vi "MCfrontPanel.vi"() -> ()   [LabVIEW 2014]
uses:
  Path.ctl
panel:
  in  "Tab Control":enum32{"Setup", "Debug", "Process", "Review"}(tab)
  in  "Next Button":bool
  in  "Previous Button":bool
  in  "Broken Path":dbl
  in  "Exceed Mirror Velocity":dbl
  in  "Number Errors":dbl
  in  "Machine":T1(tab)
  in  "Piston Controller":u16(ring) items=["Newport", "National Instruments"]
  in  "Mirrors And Laser":u16(ring) items=["Choose...", "MachineLogger", "MachineSimulator"]
  out "Bed Size":cluster{"X":dbl, "Y":dbl}
  out "MaxPower":dbl
  out "MaxSpeed":dbl
  in  "Overhand Speed (mm/s)":dbl
  in  "Mirror Speed (mm/s)":dbl
  in  "Record Images?":bool
  out "DLL_Location":path=path "C:/Users/guss2/Desktop/GVI/Git/LVslicer/MachineController/DLL"
  in  "Machine Preset":u16(ring) items=["Fraunhofer", "EOS", "Custom 1", "My Special Settings"]
  out "File":path
  out "File Stats":T2
  in  "Layer Display":dbl
  out "Yplot":dbl[](graph)
  out "Xplot":dbl[](graph)
  out "Layer":cluster{dbl[], dbl[]}(graph)
  in  "Load SCAN":bool
  in  "Beam Location":cluster{"X":dbl, "Y":dbl}
  in  "Power (W)":dbl
  in  "Laser":bool
  out "Remaining Time":string
  out "Laser Power":dbl
  out "Mirror Y":dbl
  out "Mirror X":dbl
  out "Number Errors":dbl
  out "Layer":dbl(slide) scale=0.0..1036.0
  out "3D Picture":refnum<vi>(3d-picture)
  out "ETA":timestamp
  out "Log":string
  in  "Stop Button":bool
  in  "Pause Button":bool
  in  "Play Button":bool
  out "Elapsed Time":string
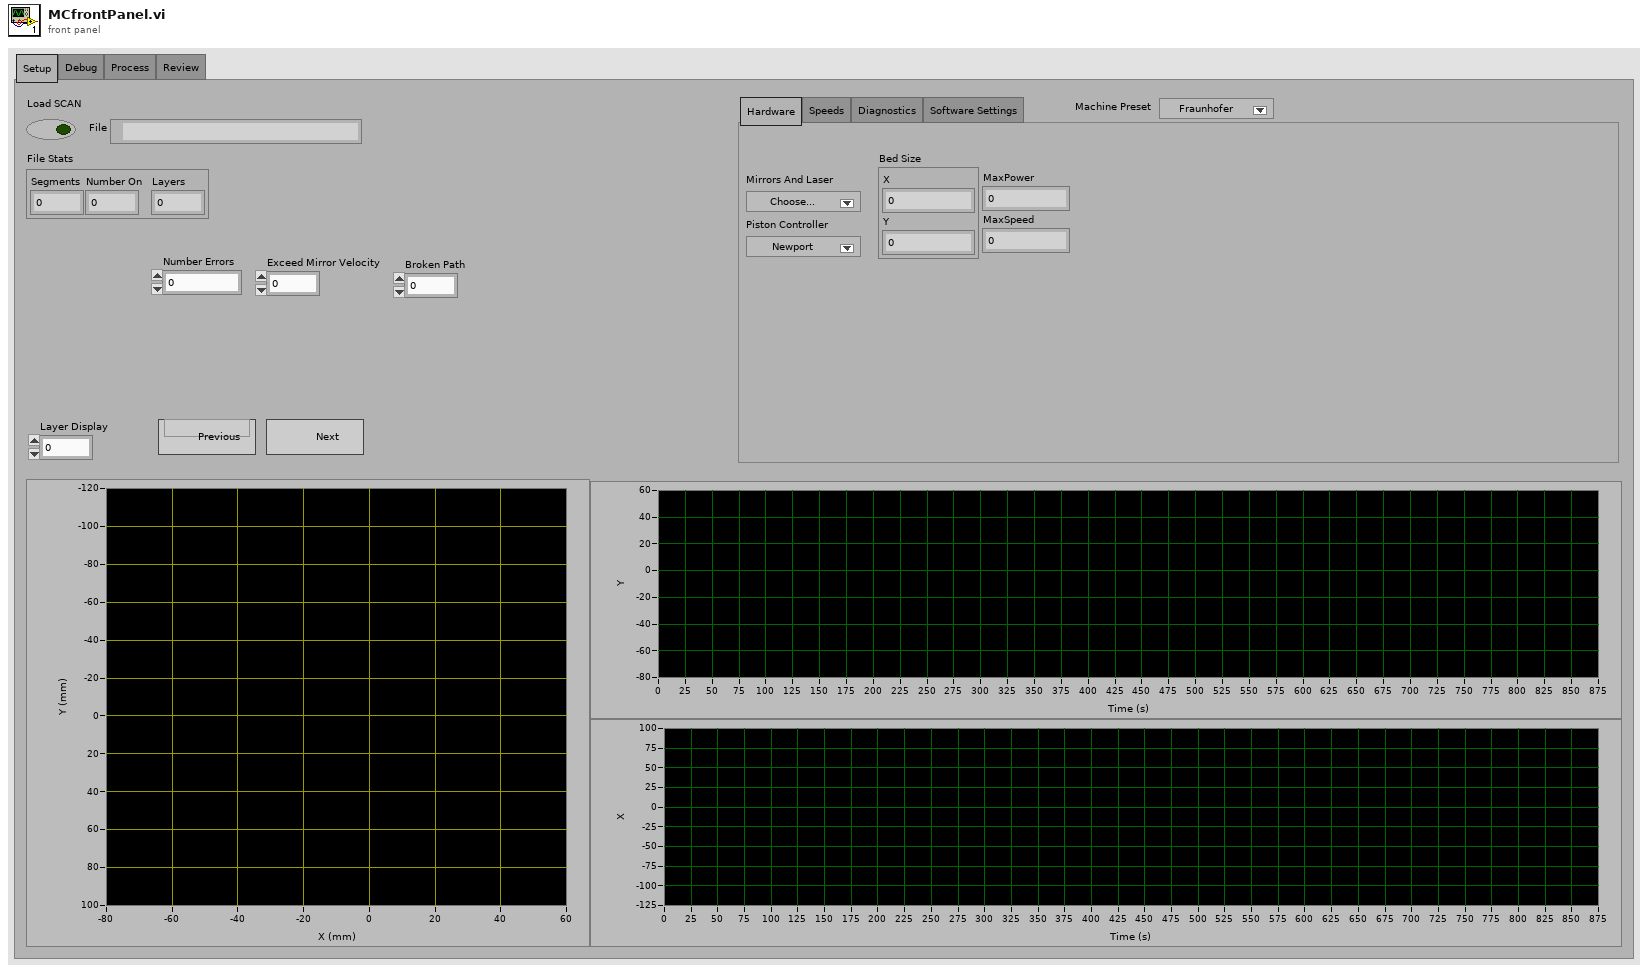
[diagram p1: front panel]
types:
  T1 = enum32{"Hardware", "Speeds", "Diagnostics", "Software Settings"}
  T2 = cluster{"Segments":dbl, "Number On":dbl, "Layers":dbl}
  T3 = typedef "Path.ctl" = cluster{"X":dbl, "Y":dbl, "OnOff":bool}[]
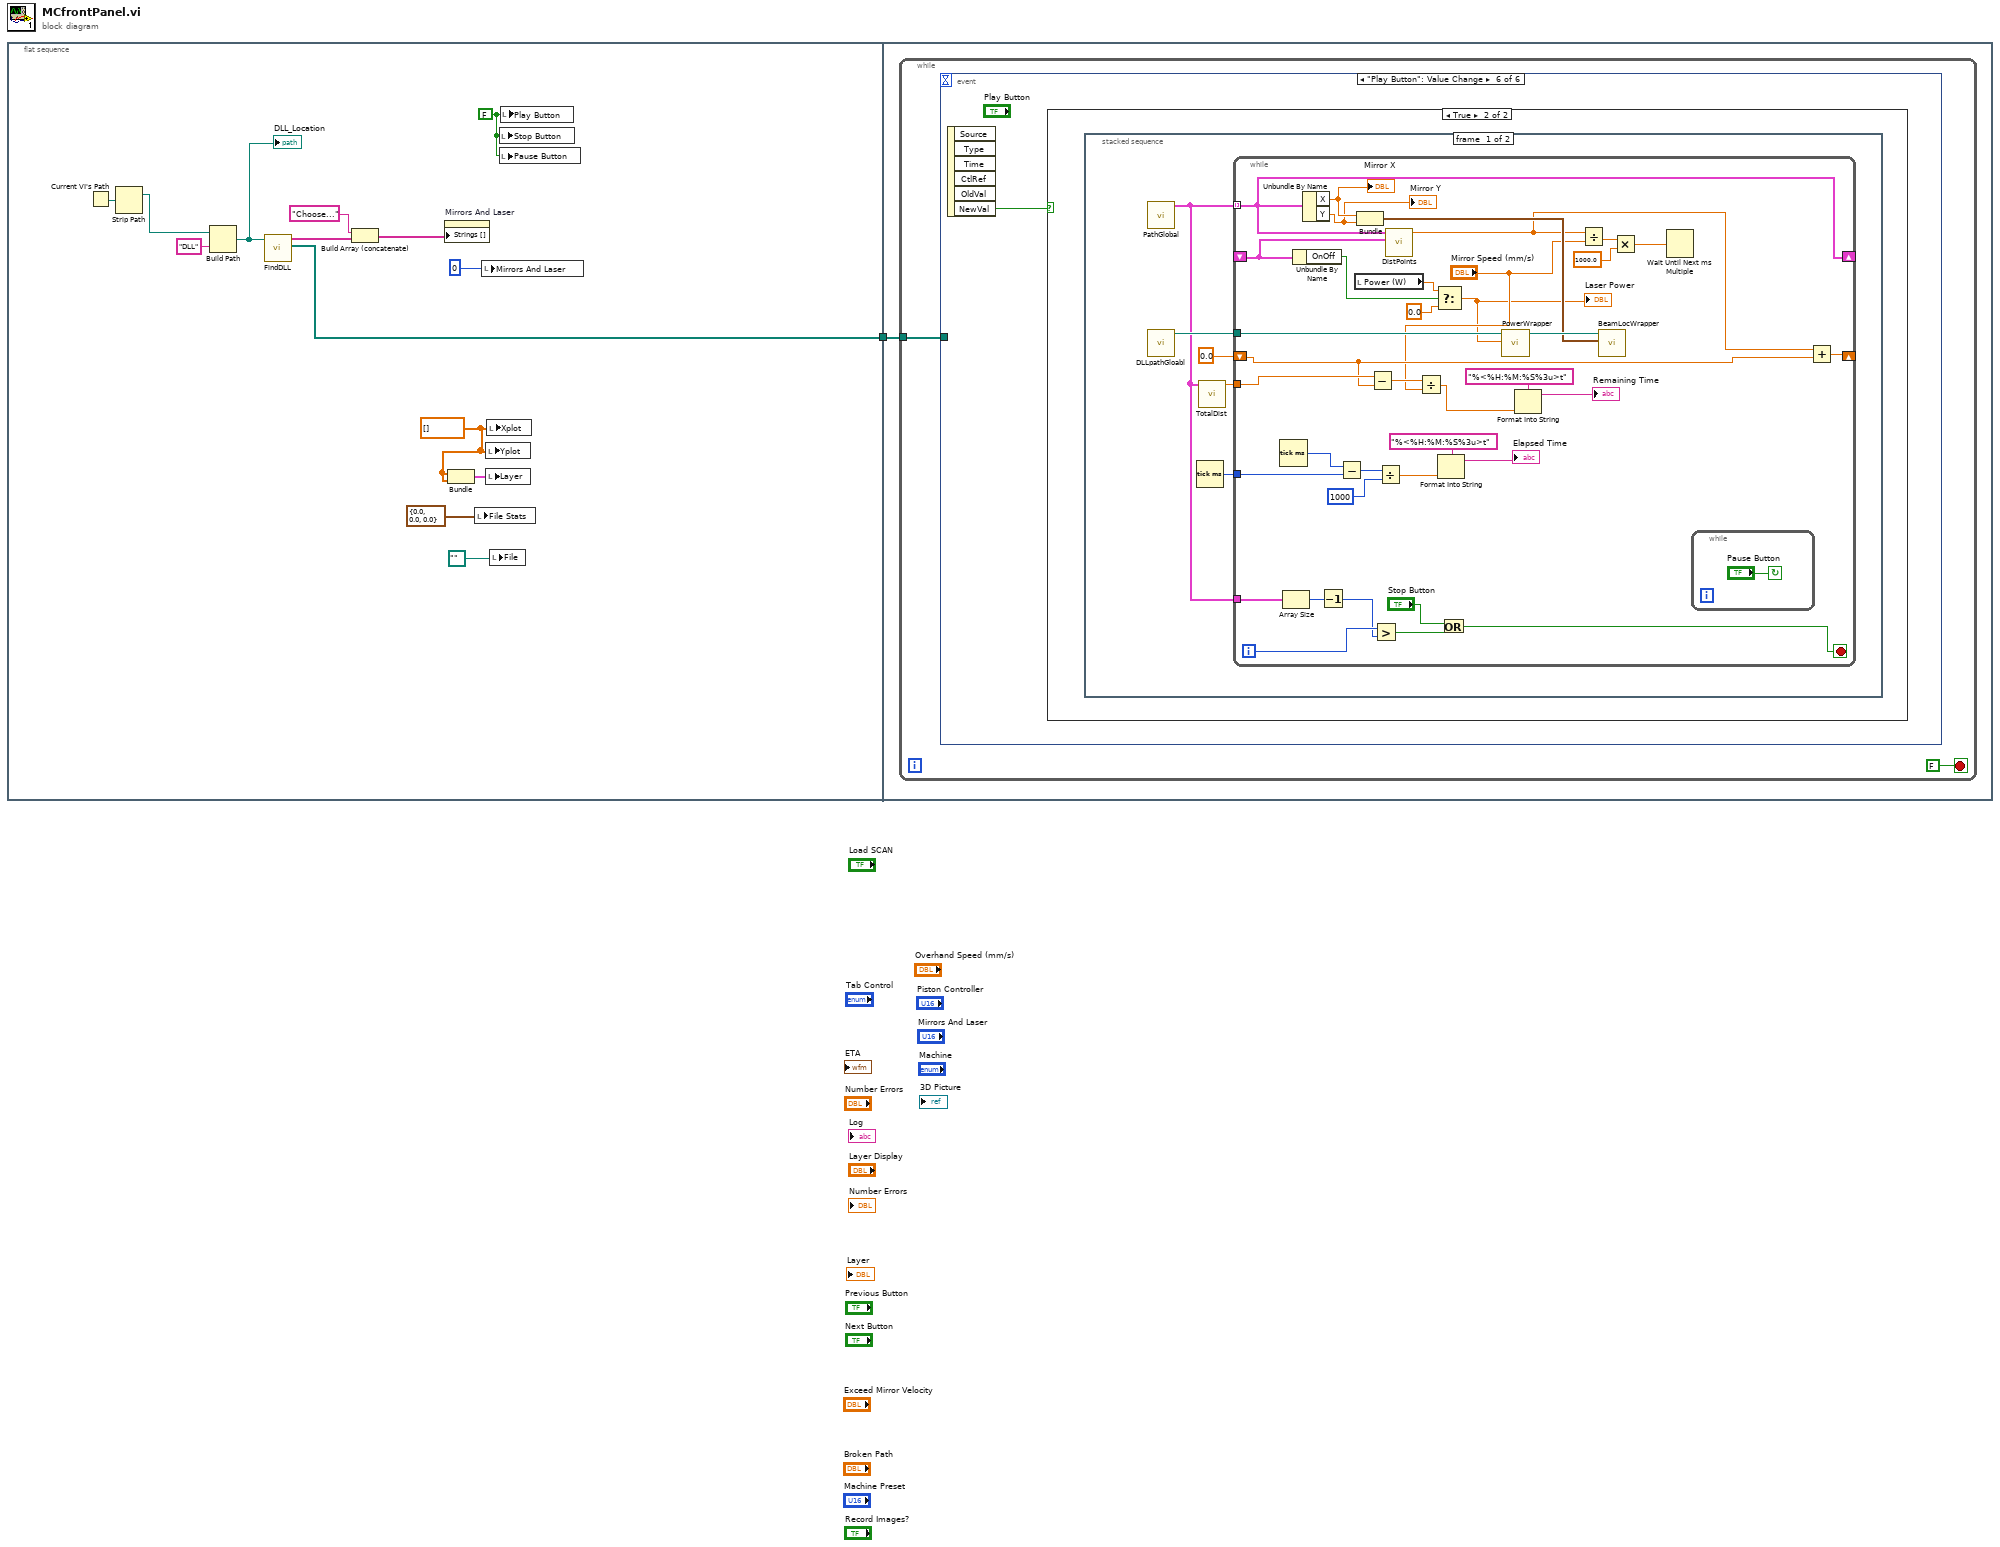
[diagram p0: block diagram]
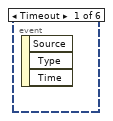
[diagram p2: hidden frame]
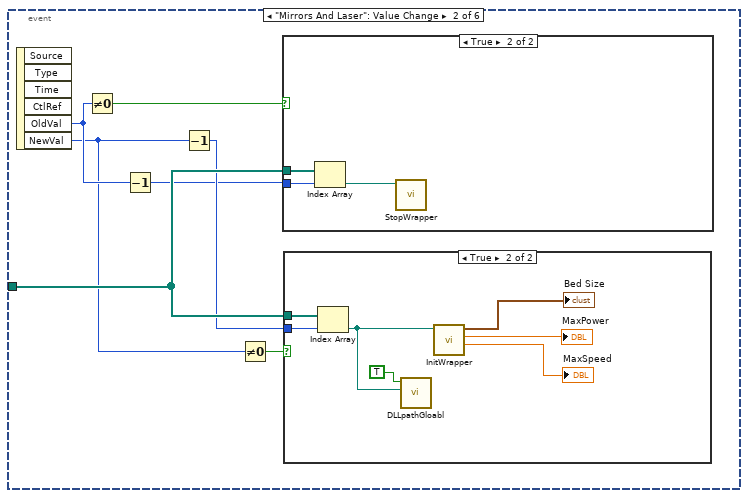
[diagram p3: hidden frame]
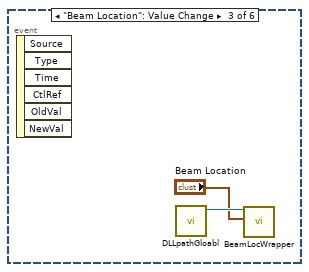
[diagram p6: hidden frame]
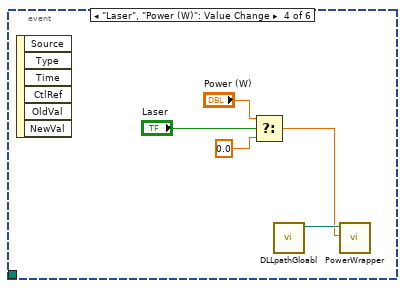
[diagram p7: hidden frame]
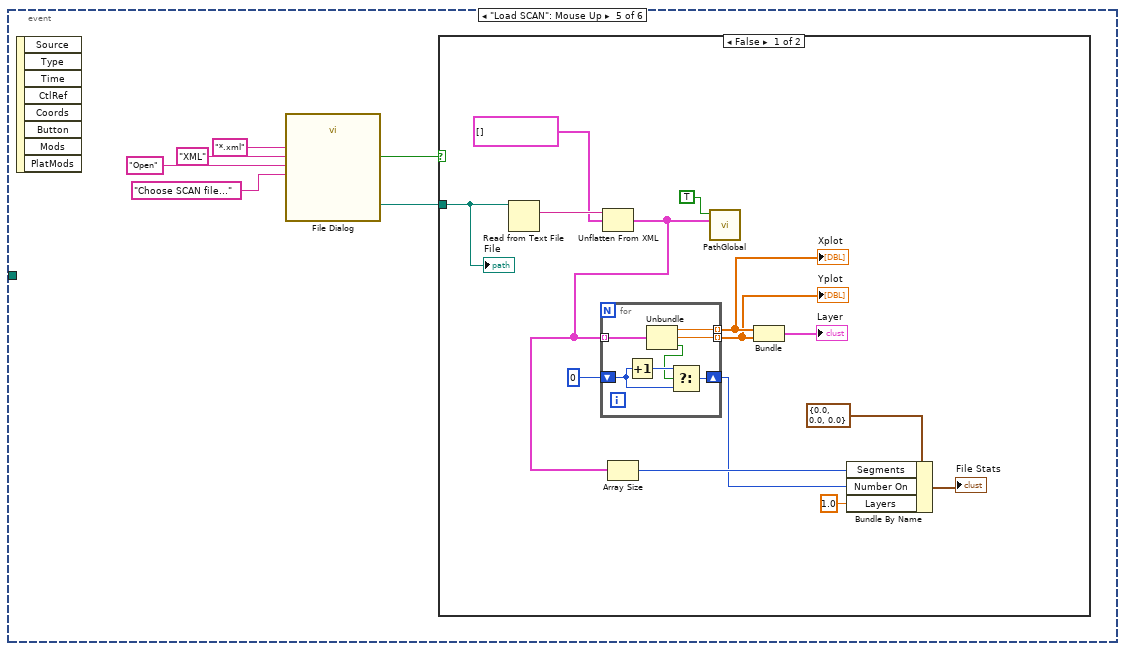
[diagram p8: hidden frame]
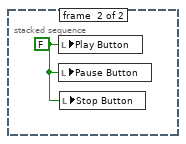
[diagram p11: hidden frame]
diagram:
  n1 = flat-sequence {
    tunnel: [w11] -> w1
    tunnel: w1 -> [w16]
    frame #0 {
      w9 = dbl[] [] ("Xplot")
      w10 = FALSE ("Play Button")
      n2 = Current VI's Path() -> (path=w3:path)
      n3 = Strip Path(path=w3) -> (stripped path=w2:path)  [unwired: 1 out]
      n4 = Build Path(base path=w2, name or relative path="DLL") -> (appended path=w4:path)
      "DLL_Location" <- w4
      n5 = call "FindDLL.vi"("DLL_Location"=w4) -> ("DLLfilepaths"=w11:path[], "DLLnames"=w14:string[])  [unwired: 9 in]
      n6 = Build Array (concatenate)("Choose..." ("filename without extension"), w14) -> (w13:string[])
      n7 = property on="Mirrors And Laser" class="Ring (strict)"("Strings []"=w13) -> ()  [unwired: 2 in, 2 out]
      n8 = Bundle("Xplot"=w9, "Xplot"=w9) -> (w8:cluster{"Xplot":dbl[], "Xplot":dbl[]})  [unwired: 1 in]
      n9 = local write "File Stats"(T2 {"Segments"=0.0, "Number On"=0.0, "Layers"=0.0} ("File Stats")) -> ()
      n10 = local write "Mirrors And Laser"(0) -> ()
      n11 = local write "Yplot"(w9) -> ()
      n12 = local write "Layer"(w8) -> ()
      n13 = local write "Xplot"(w9) -> ()
      n14 = local write "File"(path "" ("File")) -> ()
      n15 = local write "Stop Button"(w10) -> ()
      n16 = local write "Pause Button"(w10) -> ()
      n17 = local write "Play Button"(w10) -> ()
    }
    frame #1 {
      n18 = while {
        tunnel: w16 -> [w17]
        stop <- FALSE stop-if-true
        n19 = event shown="[5] \"Play Button\": Value Change" {
          selector: _ -> [_ _ _ _ _ _]
          dyn-events: _ -> [_ _ _ _ _ _]
          timeout: _ -> [_ _ _ _ _ _]
          tunnel: w17 -> [_ w24 _ _ _ _]
          event Timeout {
            n20 = event-data() -> ()  [unwired: 1 in, 3 out]
          }
          event "Mirrors And Laser": Value Change {
            n21 = event-data() -> ("OldVal"=w21:u16, "NewVal"=w19:u16)  [unwired: 1 in, 4 out]
            n22 = Not Equal To 0?(x=w21) -> (x != 0?=w25:bool)
            n23 = Decrement(x=w21) -> (x-1=w20:u16)
            n24 = Decrement(x=w19) -> (x-1=w22:u16)
            n25 = Not Equal To 0?(x=w19) -> (x != 0?=w23:bool)
            n26 = case shown="True" w25 {
              tunnel: w24 -> [_ w35]
              tunnel: w20 -> [_ w34]
              frame False {
              }
              frame True {
                n27 = Index Array(array=w35, index=w34) -> (element=w33:path)
                n28 = call "StopWrapper.vi"("DLLpath"=w33) -> ()  [unwired: 11 in]
              }
            }
            n29 = case shown="True" w23 {
              tunnel: w22 -> [_ w32]
              tunnel: w24 -> [_ w28]
              frame False {
              }
              frame True {
                n30 = Index Array(array=w28, index=w32) -> (element=w26:path)
                n31 = call "DLLpathGloabl.vi"("DLLpath"=w26, "Set/Get"=TRUE) -> ()  [unwired: 9 in, 1 out]
                n32 = call "InitWrapper.vi"("DLLpath"=w26) -> ("MaxSpeed"=→"MaxSpeed":dbl, "MaxPower"=→"MaxPower":dbl, "Bed Size"=→"Bed Size":cluster{"X":dbl, "Y":dbl})  [unwired: 8 in]
              }
            }
          }
          event "Beam Location": Value Change {
            n33 = event-data() -> ()  [unwired: 1 in, 6 out]
            n34 = call "DLLpathGloabl.vi"() -> ("PathOut"=w37:path)  [unwired: 11 in]
            n35 = call "BeamLocWrapper.vi"("Beam Location"="Beam Location", "DLLpath"=w37) -> ()  [unwired: 10 in]
          }
          event "Laser", "Power (W)": Value Change {
            n36 = event-data() -> ()  [unwired: 1 in, 6 out]
            n37 = Select(t="Power (W)", s="Laser", f=0.0) -> (s? t:f=w41:dbl)
            n38 = call "DLLpathGloabl.vi"() -> ("PathOut"=w42:path)  [unwired: 11 in]
            n39 = call "PowerWrapper.vi"("Power"=w41, "DLLpath"=w42) -> ()  [unwired: 9 in, 1 out]
          }
          event "Load SCAN": Mouse Up {
            n40 = event-data() -> ()  [unwired: 1 in, 8 out]
            n41 = call "File Dialog"("prompt"="Choose SCAN file...", "button label"="Open", "pattern (all files)"="*.xml", "pattern label"="XML") -> ("selected path"=w43:path, "cancelled"=w44:bool)  [unwired: 8 in, 2 out]
            n42 = case shown="False" w44 {
              tunnel: w43 -> [w58 _]
              frame False {
                n43 = Read from Text File(file (use dialog)=w58) -> (text=w62:string)  [unwired: 3 in, 3 out]
                n44 = Unflatten From XML(xml string=w62, type=T3 [] ("PathOut")) -> (value=w56:T3)  [unwired: 1 in, 1 out]
                n45 = for {
                  tunnel: w56 -> [w69] mode=indexing
                  tunnel: [w68] -> w50 mode=indexing
                  tunnel: [w67] -> w49 mode=indexing
                  shift-right: [w66] -> w52
                  shift-left: 0 -> [w64]
                  n46 = Increment(x=w64) -> (x+1=w65:i32)
                  n47 = Unbundle(w69) -> ("X"=w68:dbl, "Y"=w67:dbl, "OnOff"=w63:bool)
                  n48 = Select(t=w65, s=w63, f=w64) -> (s? t:f=w66:i32)
                }
                "Xplot" <- w50
                "Yplot" <- w49
                n49 = Array Size(array=w56) -> (size(s)=w53:i32)
                n50 = call "PathGlobal.vi"("Path"=w56, "Set/Get"=TRUE) -> ()  [unwired: 9 in, 1 out]
                n51 = Bundle(w50, w49) -> (→"Layer":cluster{dbl[], dbl[]})  [unwired: 1 in]
                n52 = Bundle By Name(cluster=T2 {"Segments"=0.0, "Number On"=0.0, "Layers"=0.0} ("File Stats"), "Segments"=w53, "Number On"=w52, "Layers"=1.0) -> (→"File Stats":T2)
                "File" <- w58
              }
              frame True {
              }
            }
          }
          event "Play Button": Value Change {
            n53 = event-data() -> ("NewVal"=w70:bool)  [unwired: 1 in, 5 out]
            n54 = case shown="True" w70 {
              frame False {
              }
              frame True {
                n55 = stacked-sequence {
                  frame #0 {
                    n56 = call "PathGlobal.vi"() -> ("PathOut"=w74:T3)  [unwired: 11 in]
                    n57 = call "DLLpathGloabl.vi"() -> ("PathOut"=w75:path)  [unwired: 11 in]
                    n58 = Tick Count (ms)() -> (millisecond timer value=w73:u32)
                    n59 = call "TotalDist.vi"("Path"=w74) -> ("TotalDistance"=w72:dbl)  [unwired: 10 in]
                    n60 = while {
                      tunnel: w74 -> [w96] mode=indexing
                      tunnel: w74 -> [w112]
                      shift-right: [w96] -> _
                      shift-left: _ -> [w95]
                      tunnel: w75 -> [w103]
                      tunnel: w73 -> [w93]
                      tunnel: w72 -> [w85]
                      shift-right: [w87] -> _
                      shift-left: 0.0 -> [w84]
                      i -> [w111]
                      stop <- w106 stop-if-true
                      n61 = Tick Count (ms)() -> (millisecond timer value=w94:u32)
                      n62 = Array Size(array=w112) -> (size(s)=w109:i32)
                      n63 = Unbundle By Name(w95) -> ("OnOff"=w97:bool)
                      n64 = Unbundle By Name(w96) -> ("X"=w78:dbl, "Y"=w77:dbl)
                      "Mirror X" <- w78
                      "Mirror Y" <- w77
                      n65 = Decrement(x=w109) -> (x-1=w108:i32)
                      n66 = Subtract(x=w94, y=w93) -> (x-y=w91:u32)
                      n67 = local read "Power (W)"() -> (w105:dbl)
                      n68 = Bundle("X"=w78, "Y"=w77) -> (w101:cluster{"X":dbl, "Y":dbl})  [unwired: 1 in]
                      n69 = Subtract(x=w85, y=w84) -> (x-y=w83:dbl)
                      n70 = Greater?(x=w111, y=w108) -> (0:w110:bool)
                      n71 = Divide(x=w91, y=u32 1000) -> (x/y=w88:dbl)
                      n72 = call "DistPoints.vi"("Point2"=w95, "Point1"=w96) -> ("Distance"=w86:dbl)  [unwired: 9 in]
                      n73 = Divide(x=w83, y="Mirror Speed (mm/s)") -> (x/y=w80:dbl)
                      n74 = Select(t=w105, s=w97, f=0.0) -> (s? t:f=w76:dbl)
                      "Laser Power" <- w76
                      n75 = Format Into String(format string="%<%H:%M:%S%3u>t", w88) -> (resulting string=→"Elapsed Time":string)  [unwired: 2 in, 1 out]
                      n76 = Or(x="Stop Button", y=w110) -> (x .or. y?=w106:bool)
                      n77 = call "PowerWrapper.vi"("Power"=w76, "DLLpath"=w103) -> ("DLLpathOUt"=w102:path)  [unwired: 9 in]
                      n78 = Format Into String(format string="%<%H:%M:%S%3u>t", w80) -> (resulting string=→"Remaining Time":string)  [unwired: 2 in, 1 out]
                      n79 = Divide(x=w86, y="Mirror Speed (mm/s)") -> (x/y=w100:dbl)
                      n80 = call "BeamLocWrapper.vi"("Beam Location"=w101, "DLLpath"=w102) -> ()  [unwired: 10 in]
                      n81 = Multiply(x=w100, y=1000.0) -> (x*y=w98:dbl)
                      n82 = Wait Until Next ms Multiple(millisecond multiple=w98) -> ()  [unwired: 1 out]
                      n83 = while {
                        stop <- "Pause Button" continue-if-true
                      }
                      n84 = Add(x=w86, y=w84) -> (x+y=w87:dbl)
                    }
                  }
                  frame #1 {
                    w114 = FALSE ("Play Button")
                    n85 = local write "Play Button"(w114) -> ()
                    n86 = local write "Pause Button"(w114) -> ()
                    n87 = local write "Stop Button"(w114) -> ()
                  }
                }
              }
            }
          }
        }
      }
    }
  }
